vi "sv_Swept Settling Time to Samples.vi"(6 "settling time":cluster{"settle time":dbl, "settle cycles":i32} {"settle time" format="%.2f"}, 7 "frequency to generate [Hz]":dbl format="%.2f", 10 "AI sampling frequency":dbl format="%.2f", 11 "indice computations in":T1) -> (2 "dup AI sampling frequency":dbl format="%.2f", 3 "indice computations in":T1)   [LabVIEW 2017, in "SoundVib_SweptSine.lvlib"]
uses:
  <vilib>/addons/Sound and Vibration/svt_Swept Sine/SoundVib_SweptSine.lvlib
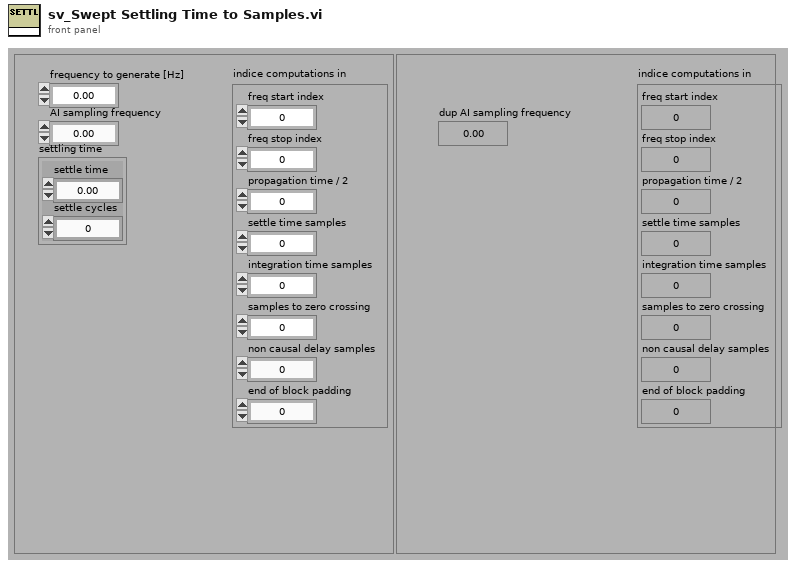
[diagram p1: front panel]
types:
  T1 = cluster{"freq start index":u32, "freq stop index":u32, "propagation time / 2":u32, "settle time samples":u32, "integration time samples":u32, "samples to zero crossing":u32, "non causal delay samples":u32, "end of block padding":u32}
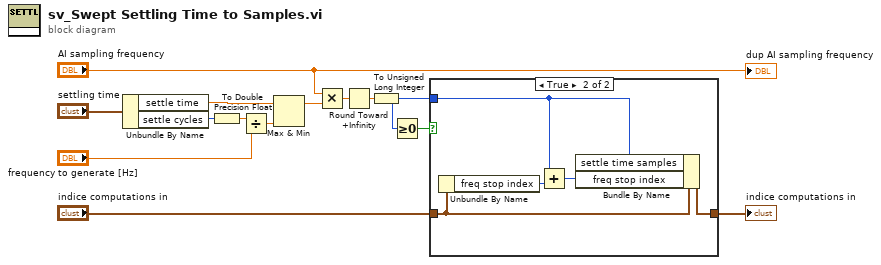
[diagram p0: block diagram]
diagram:
  n1 = Unbundle By Name("settling time") -> ("settle time"=w7:dbl, "settle cycles"=w5:i32)
  n2 = To Double Precision Float(number=w5) -> (double precision float=w13:dbl)
  n3 = Divide(x=w13, y="frequency to generate [Hz]") -> (x/y=w12:dbl)
  n4 = Max & Min(x=w7, y=w12) -> (max(x,y)=w10:dbl)  [unwired: 1 out]
  n5 = Multiply(x="AI sampling frequency", y=w10) -> (x*y=w11:dbl)
  n6 = Round Toward +Infinity(x=w11) -> (ceil(x): smallest int >= x=w9:dbl)
  n7 = To Unsigned Long Integer(number=w9) -> (unsigned 32bit integer=w2:u32)
  n8 = Greater Or Equal To 0?(x=w2) -> (x >= 0?=w1:bool)
  n9 = case shown="True" w1 {
    tunnel: [w15 w20] -> w4
    tunnel: "indice computations in" -> [w15 w19]
    tunnel: w2 -> [_ w16]
    frame False {
    }
    frame True {
      n10 = Unbundle By Name(w19) -> ("freq stop index"=w18:u32)
      n11 = Add(x=w16, y=w18) -> (x+y=w17:u32)
      n12 = Bundle By Name(cluster=w19, "settle time samples"=w16, "freq stop index"=w17) -> (w20:T1)
    }
  }
  "indice computations in" <- w4
  "dup AI sampling frequency" <- "AI sampling frequency"
